vi "send&receive_img-tmp.vi"() -> ()   [LabVIEW 2018]
uses:
  Server or client state.ctl
  detailed error info.ctl
  StackFrame.ctl
  Commands.ctl
  21ea884c-855a-42e1-a4b3-29a64fa611ff.vi
  21ea884c-855a-42e1-a4b3-29a64fa611ff.vi/e3bd8dab-eb54-4af8-8972-953366dfaab9.vi
  21ea884c-855a-42e1-a4b3-29a64fa611ff.vi/e3bd8dab-eb54-4af8-8972-953366dfaab9.vi/6ffe13b8-d26a-4ba7-8790-9bb9c8f67003.vi
  21ea884c-855a-42e1-a4b3-29a64fa611ff.vi/e3bd8dab-eb54-4af8-8972-953366dfaab9.vi/6b80f738-d5b8-4f0a-a577-af0b5cf050b5.vi
  21ea884c-855a-42e1-a4b3-29a64fa611ff.vi/e3bd8dab-eb54-4af8-8972-953366dfaab9.vi/8fa79093-f932-45fa-9128-458e5b3adbca.vi
  jl-scripts path.vi
  <vilib>/Utility/error.llb/Error Cluster From Error Code.vi
  check ID validity.vi
  bindata_descr to JSON.vi
  check cluster field names.vi
  concat JSON.vi
  build request.vi
  Parse server response.vi
  log jl exceptions.vi
  <vilib>/ErrorRing/Error Ring.xnode
  LV-0mq-Julia_roundtrip-lib.lvlib
panel:
  in  "go":bool caption="go (Julia Server started externally)"
  in  "Start with Julia":bool caption="Start Julia Server and go"
  out "ZMQ timeout":bool
  out "picture dup":picture
  in  "peppers":bool
  in  "Path":path=path "C:/_MyOwnDocs/MyTmp/ScreenShots/2019-07-30 14_38_29-Desktop Execution Trace Toolkit.png"
  out "picture":picture
  in  "next":bool
  in  "stop LV only":bool
  in  "stop":bool
  out "detailed error info":T1
  out "Jl Server state out":T3
  out "short err code":u8
  out "final error":errorcluster
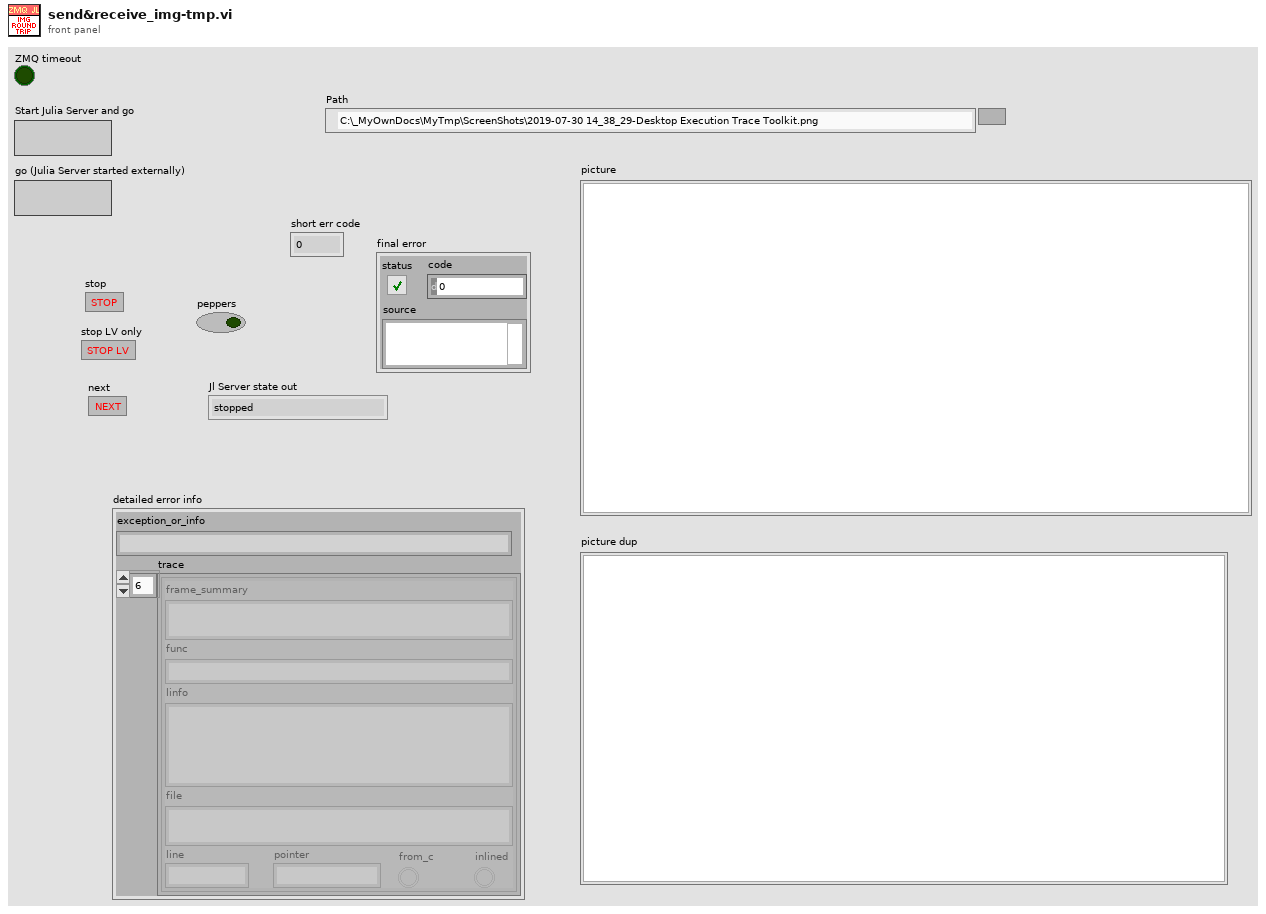
[diagram p1: front panel]
types:
  T1 = typedef "LV-0mq-Julia_roundtrip-lib.lvlib/detailed error info.ctl" = cluster{"exception_or_info":string, "trace":T2[]}
  T2 = typedef "LV-0mq-Julia_roundtrip-lib.lvlib/StackFrame.ctl" = cluster{"frame_summary":string, "func":string, "linfo":string, "file":string, "line":i32, "pointer":u64, "from_c":bool, "inlined":bool}
  T3 = typedef "LV-0mq-Julia_roundtrip-lib.lvlib/Server or client state.ctl" = enum16{"stopped", "running", "unknown"}
  T4 = typedef "LV-0mq-Julia_roundtrip-lib.lvlib/Commands.ctl" = enum16{"Start Jl-server & Init LV-client", "Send request & Get response ", "Stop Jl-server & Cleanup LV-client", "Cleanup LV-client", "Start Jl-server", "Stop Jl-server", "Init LV-Client", "Cleanup LV-Client", "(not allowed)", "Set LV Client state", "Set Jl Server state", "set ZMQ timeout", "read ZMQ timeout", "read-out state"}
  T5 = typedef "imagedata.ctl" = cluster{"image type":i32, "image depth":i32, "image":u8[], "mask":u8[], "colors":u32[], "Rectangle":cluster{"left":i16, "top":i16, "right":i16, "bottom":i16}}
  T6 = typedef "LV-0mq-Julia_roundtrip-lib.lvlib/Bindata&description.ctl" = cluster{"bindata_descr":T7[], "bindata":u8[]}
  T7 = typedef "LV-0mq-Julia_roundtrip-lib.lvlib/Bindata description.ctl" = cluster{"nofbytes":i32, "numtype":string, "start":i32, "arrdims":i32[], "kwarg_name":string, "category":string}
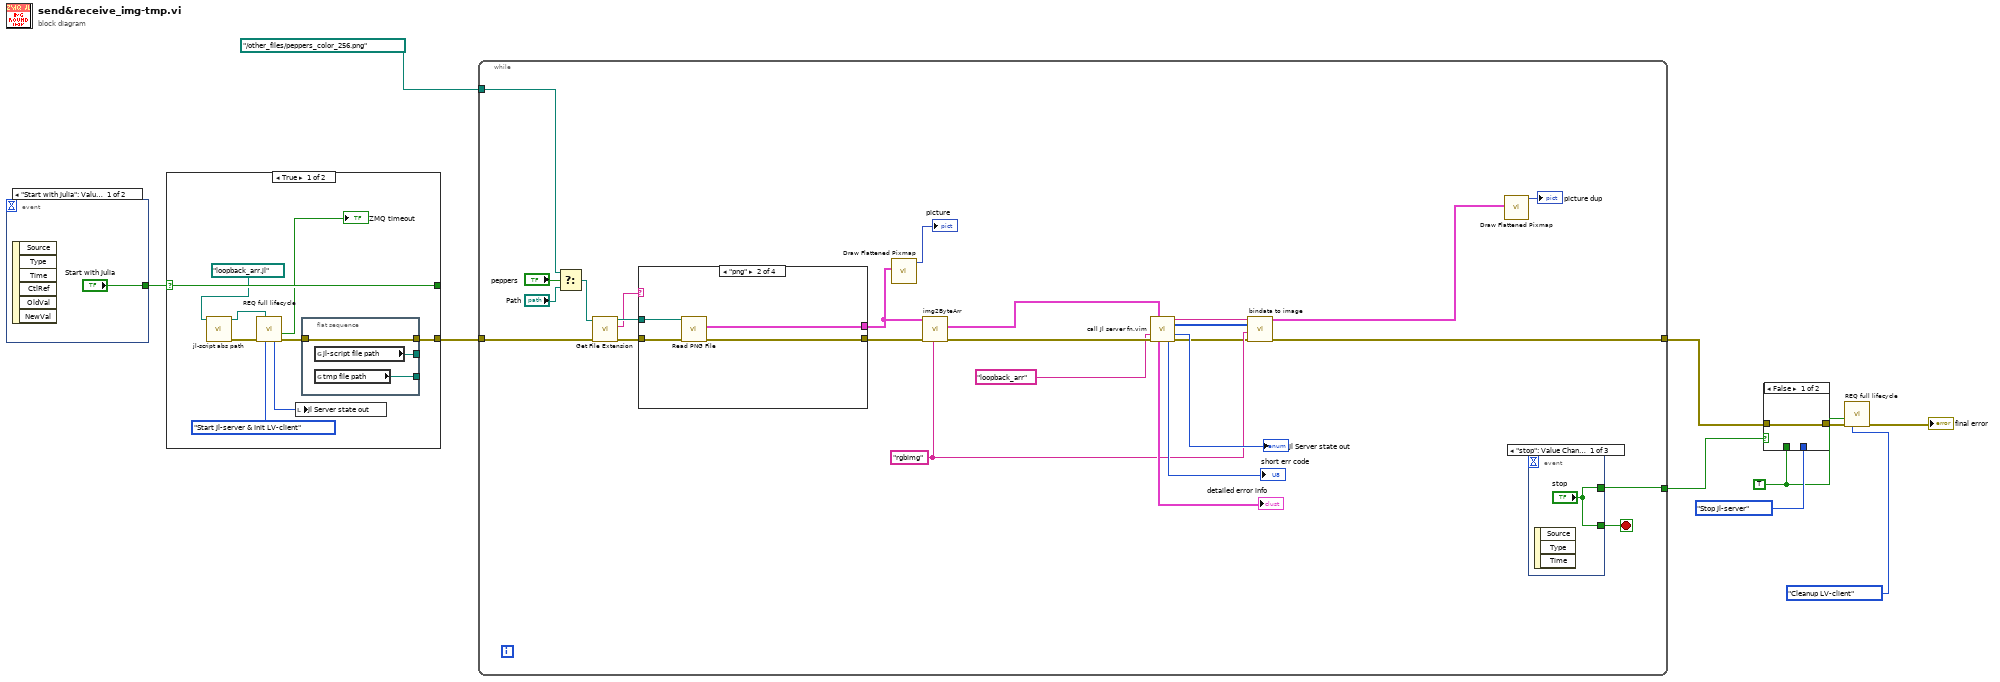
[diagram p0: block diagram]
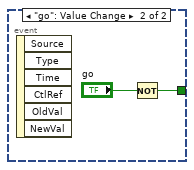
[diagram p2: hidden frame]
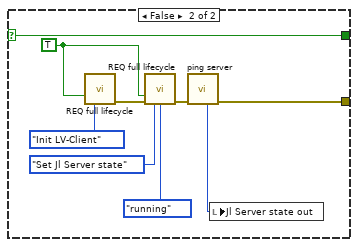
[diagram p3: hidden frame]
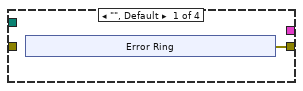
[diagram p4: hidden frame]
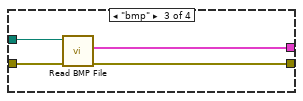
[diagram p5: hidden frame]
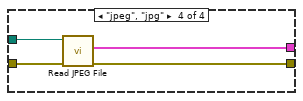
[diagram p6: hidden frame]
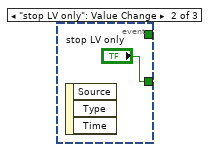
[diagram p7: hidden frame]
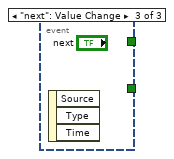
[diagram p8: hidden frame]
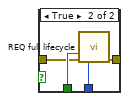
[diagram p9: hidden frame]
diagram:
  w6 = TRUE ("Force command")
  n1 = event shown="[0] \"Start with Julia\": Value Change" {
    selector: _ -> [_ _]
    dyn-events: _ -> [_ _]
    timeout: _ -> [_ _]
    tunnel: ["Start with Julia" w12] -> w2
    event "Start with Julia": Value Change {
      n2 = event-data() -> ()  [unwired: 1 in, 6 out]
    }
    event "go": Value Change {
      n3 = event-data() -> ()  [unwired: 1 in, 6 out]
      n4 = Not(x="go") -> (.not. x?=w12:bool)
    }
  }
  n5 = case shown="True" w2 {
    selector: w2 -> [w21 w30]
    tunnel: [w18 w26] -> w1
    tunnel: [w21 w30] -> _
    frame True {
      n6 = call "jl-script abs path.vi"("Julia user functions script"=path "loopback_arr.jl") -> ("error out"=w16:errorcluster, "script abs path"=w17:path)  [unwired: 9 in]
      n7 = call "REQ full lifecycle.vi"("Julia user functions script"=w17, "error in"=w16, "command"=Commands."Start Jl-server & Init LV-client") -> ("timeout?"=→"ZMQ timeout":bool, "Jl Server state out"=w20:T3, "error out"=w19:errorcluster)  [unwired: 6 in, 4 out]
      n8 = local write "Jl Server state out"(w20) -> ()
      n9 = flat-sequence {
        tunnel: [w25] -> w18
        tunnel: w19 -> [w25]
        tunnel: [w24] -> _
        tunnel: [w23] -> _
        frame #0 {
          n10 = global read "jl-scripts path.vi" "jl-script file path"() -> (w24:path)
          n11 = global read "jl-scripts path.vi" "tmp file path"() -> (w23:path)
        }
      }
    }
    frame False {
      w32 = TRUE ("Force command")
      n12 = call "REQ full lifecycle.vi"("Force command"=w32, "command"=Commands."Init LV-Client") -> ("error out"=w29:errorcluster)  [unwired: 7 in, 6 out]
      n13 = call "REQ full lifecycle.vi"("Force command"=w32, "error in"=w29, "command"=Commands."Set Jl Server state", "Jl Server state in"=Server_or_client_state."running") -> ("error out"=w28:errorcluster)  [unwired: 5 in, 6 out]
      n14 = call "ping server.vi"("error in"=w28) -> ("error out"=w26:errorcluster, "Jl Server state out"=w27:T3)  [unwired: 6 in, 3 out]
      n15 = local write "Jl Server state out"(w27) -> ()
    }
  }
  n16 = while {
    tunnel: w1 -> [w40]
    tunnel: [w59] -> w5
    tunnel: path "../other_files/peppers_color_256.png" ("Path") -> [w55]
    tunnel: [w41] -> w3
    stop <- w60 stop-if-true
    w44 = "rgbimg" ("Tag")
    n17 = Select(t=w55, s="peppers", f="Path") -> (s? t:f=w39:path)
    n18 = call <vilib>:"Get File Extension.vi"("error in (no error)"=w40, "file"=w39) -> ("error out"=w37:errorcluster, "lowercase file extension"=w35:string, "dup file"=w38:path)  [unwired: 5 in, 2 out]
    n19 = case shown="\"png\"" w35 {
      tunnel: [_ w70 w74 w78] -> w53
      tunnel: w38 -> [_ w69 w73 w77]
      tunnel: w37 -> [_ w68 w72 w76]
      tunnel: [w61 w67 w71 w75] -> w36
      frame "", Default {
        n20 = xnode "Error Ring"() -> ("error out"=w61:errorcluster)
      }
      frame "png" {
        n21 = call <vilib>:"Read PNG File.vi"("error in (no error)"=w68, "path to PNG file"=w69) -> ("error out"=w67:errorcluster, "image data"=w70:T5)  [unwired: 7 in, 1 out]
      }
      frame "bmp" {
        n22 = call <vilib>:"Read BMP File.vi"("error in (no error)"=w72, "path to BMP file"=w73) -> ("error out"=w71:errorcluster, "image data"=w74:T5)  [unwired: 7 in, 1 out]
      }
      frame "jpeg", "jpg" {
        n23 = call <vilib>:"Read JPEG File.vi"("error in (no error)"=w76, "path to JPEG file"=w77) -> ("error out"=w75:errorcluster, "image data"=w78:T5)  [unwired: 7 in, 1 out]
      }
    }
    n24 = call <vilib>:"Draw Flattened Pixmap.vi"("image data"=w53) -> ("new picture"=→"picture":picture)  [unwired: 8 in]
    n25 = call "img2ByteArr.vi"("kwarg_name"=w44, "error in (no error)"=w36, "img in"=w53) -> ("error out"=w49:errorcluster, "Bindata & descr out"=w47:T6)  [unwired: 6 in, 1 out]
    n26 = call "call Jl server fn.vim"("Bindata & descr in"=w47, "fun2call"="loopback_arr", "error in (no error)"=w49) -> ("JSON received"=w46:string, "binary data received"=w45:u8[], "Jl Server state out"=→"Jl Server state out":T3, "detailed error info"=→"detailed error info":T1, "return code"=→"short err code":u8, "error out"=w42:errorcluster)  [unwired: 6 in, 1 out]
    n27 = call "bindata to image.vi"("error in (no error)"=w42, "name"=w44, "binary data in"=w45, "JSON in"=w46) -> ("error out"=w41:errorcluster, "img out"=w43:T5)  [unwired: 6 in]
    n28 = call <vilib>:"Draw Flattened Pixmap.vi"("image data"=w43) -> ("new picture"=→"picture dup":picture)  [unwired: 8 in]
    n29 = event shown="[0] \"stop\": Value Change" {
      selector: _ -> [_ _ _]
      dyn-events: _ -> [_ _ _]
      timeout: _ -> [_ _ _]
      tunnel: ["stop" "stop LV only" _] -> w60
      tunnel: ["stop" _ _] -> w59
      event "stop": Value Change {
        n30 = event-data() -> ()  [unwired: 1 in, 3 out]
      }
      event "stop LV only": Value Change {
        n31 = event-data() -> ()  [unwired: 1 in, 3 out]
      }
      event "next": Value Change {
        n32 = event-data() -> ()  [unwired: 1 in, 3 out]
      }
    }
  }
  n33 = case shown="False" w5 {
    tunnel: Commands."Stop Jl-server" ("command") -> [_ w85]
    tunnel: [w81 w84] -> w9
    tunnel: w6 -> [_ w83]
    tunnel: w3 -> [w81 w82]
    frame False {
    }
    frame True {
      n34 = call "REQ full lifecycle.vi"("Force command"=w83, "error in"=w82, "command"=w85) -> ("error out"=w84:errorcluster)  [unwired: 6 in, 6 out]
    }
  }
  n35 = call "REQ full lifecycle.vi"("Force command"=w6, "error in"=w9, "command"=Commands."Cleanup LV-client") -> ("error out"=→"final error":errorcluster)  [unwired: 6 in, 6 out]
